vi "Available UART.vi"(8 "error in (no error)":errorcluster, 11 "DeviceComms in":refnum<class "DeviceComms.lvclass">) -> (0 "error out":errorcluster, 2 "Available UART":T1[](array[typedef]), 3 "DeviceComms out":refnum<class "DeviceComms.lvclass">)   [LabVIEW 2020, in "CTI.lvlib" / "DeviceComms.lvclass"]
uses:
  DeviceComms.lvclass
  GPIO Number.ctl
  CTI.lvlib
  UART Number.ctl
  Available UART.ctl
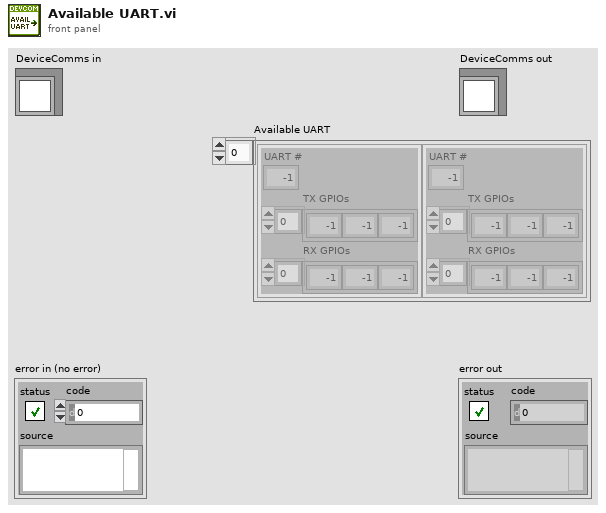
[diagram p1: front panel]
types:
  T1 = typedef "CTI.lvlib/Available UART.ctl" = cluster{"UART #":T2, "TX GPIOs":T3[], "RX GPIOs":T3[]}
  T2 = typedef "CTI.lvlib/UART Number.ctl" = i8
  T3 = typedef "CTI.lvlib/GPIO Number.ctl" = i8
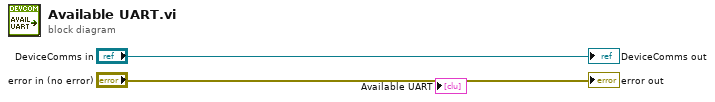
[diagram p0: block diagram]
diagram:
  "error out" <- "error in (no error)"
  "DeviceComms out" <- "DeviceComms in"
